vi "Do.vi"(8 "error in (no error)":errorcluster, 10 "Actor in":refnum<class "Actor.lvclass">, 11 "Load and Run Sequence Msg":refnum<class "Load and Run Sequence Msg.lvclass">) -> (0 "error out":errorcluster, 2 "Actor out":refnum<class "Actor.lvclass">)   [LabVIEW 2020, in "Sequencer.lvlib" / "Load and Run Sequence Msg.lvclass"]
doc: "This implementation loads and compiles a sequence and then enqueues it in front on the Sequencer Core."
uses:
  Load and Run Sequence Msg.lvclass
  C:/Current projects/WS/LV32.2020..HDH.ActorFramework.Core/Actor/Sequencer/Sequencer Messages/Sequencer Msg/Sequencer Msg.lvclass
  PPL/HDH.Actor Framework.Core.Actor.lvlibp/1abvi3w/vi.lib/ActorFramework/Actor/Actor.lvclass
  Sequencer/Sequencer.lvclass
  C:/Current projects/WS/PPL/HDH.Actor Framework.Core.Actor.lvlibp/1abvi3w/vi.lib/ActorFramework/Actor/Actor.lvclass
  Sequencer Msg/Sequencer Msg.lvclass/Sequencer Msg.ctl
  Load and Run Sequence Msg.lvclass/Load and Run Sequence Msg.ctl
  Batch Msg/Batch Msg.lvclass
  C:/Current projects/WS/PPL/HDH.Actor Framework.Core.Actor.lvlibp/1abvi3w/vi.lib/ActorFramework/Message/Message.lvclass
  Sequencer.lvlib
  Sequencer Msg/Sequencer Msg.lvclass
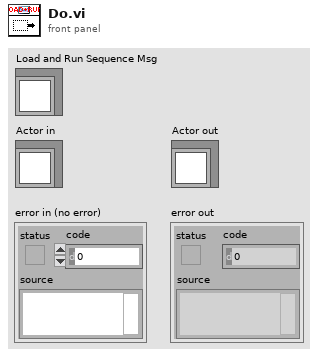
[diagram p1: front panel]
types:
  T1 = typedef "Sequencer.lvlib/Ctl_MessageListElement.ctl" = cluster{"Base Name":string, "List index":i32, "Msg path":path, "Supports DA?":bool, "Symbol":i32}
  T2 = typedef "Sequencer.lvlib/Ctl_SequenceElement.ctl" = cluster{"Message Base Name":string, "Message Path":path, "Supports Data Access?":bool, "List Symbol":i32, "Sequence Control Element Array":T3[]}
  T3 = typedef "Sequencer.lvlib/Ctl_SequenceControlElement.ctl" = cluster{"Data Override name":string, "Looped Override?":bool, "Control element":T4, "List Symbol":i32}
  T4 = typedef "HDH.Actor Framework.Core.Msg.lvlibp/Ctl_Control Element.ctl" = cluster{"Index":i32, "Label":string, "Value":variant}
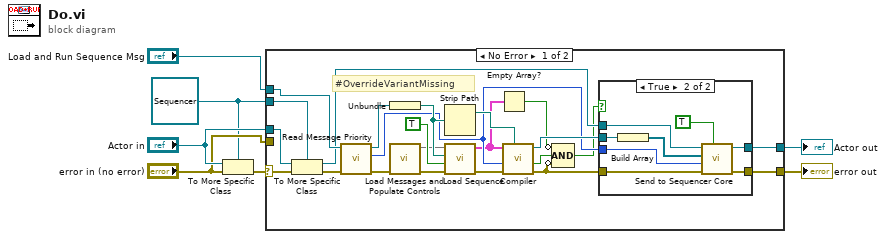
[diagram p0: block diagram]
diagram:
  w1 = refnum<class "Sequencer.lvclass"> refnum ("Sequencer.lvlib:Sequencer.lvclass")
  n1 = To More Specific Class(target class=w1, reference="Actor in", error in="error in (no error)") -> (error out=w4:errorcluster)  [unwired: 1 out]
  n2 = case shown="No Error" w4 {
    selector: w4 -> [w24 _]
    tunnel: [w17 w41] -> w7
    tunnel: [w16 w42] -> w6
    tunnel: "Actor in" -> [w22 w42]
    tunnel: "Load and Run Sequence Msg" -> [w27 _]
    tunnel: "error in (no error)" -> [_ w41]
    tunnel: w1 -> [w21 _]
    frame No Error {
      # "#OverrideVariantMissing"
      n3 = To More Specific Class(target class=w21, reference=w22, error in=w24) -> (specific class reference=w20:refnum<class "Sequencer.lvclass">, error out=w23:errorcluster)
      n4 = call "Read Message Priority.vi"("error in (no error)"=w23, "Sequencer Msg in"=w27) -> ("error out"=w10:errorcluster, "Priority"=w18:u16, "Sequencer Msg out"=w26:refnum<class "Load and Run Sequence Msg.lvclass">)  [unwired: 7 in]
      n5 = Unbundle(w26) -> (w29:path)
      n6 = call "Load Messages and Populate Controls.vi"("error in (no error)"=w10) -> ("error out"=w9:errorcluster, "Message map"=w8:map{string, T1})  [unwired: 9 in]
      n7 = Strip Path(path=w29) -> (stripped path=w28:path)  [unwired: 1 out]
      n8 = call "Load Sequence.vi"("error in (no error)"=w9, "Skip File Dialog?(F)"=TRUE, "Browse path"=w29, "Message map"=w8) -> ("error out"=w25:errorcluster, "Uncompiled Sequence out"=w15:T2[])  [unwired: 6 in]
      n9 = Empty Array?(array=w15) -> (empty?=w14:bool)
      n10 = call "Compiler.vi"("Sequence folder path"=w28, "error in (no error)"=w25, "Message Priority(Normal)"=w18, "Uncompiled sequence in"=w15) -> ("error out"=w12:errorcluster, "Success?"=w13:bool, "Batch Msg out"=w19:refnum<class "Batch Msg.lvclass">)  [unwired: 5 in]
      n11 = Compound Arithmetic op=AND(invert w14, w13, invert w12) -> (w11:bool)
      n12 = case shown="True" w11 {
        tunnel: w20 -> [w31 w40]
        tunnel: w19 -> [_ w39]
        tunnel: w18 -> [_ w36]
        tunnel: [w32 w35] -> w17
        tunnel: [w31 w34] -> w16
        tunnel: w12 -> [w32 w33]
        frame False {
        }
        frame True {
          n13 = Build Array(w39) -> (w38:refnum<class "Batch Msg.lvclass">[])
          n14 = call "Send to Sequencer Core.vi"("In Front?(F)"=TRUE, "error in (no error)"=w33, "Message Priority"=w36, "Message Array"=w38, "Sequencer in"=w40) -> ("error out"=w35:errorcluster, "Sequencer out"=w34:refnum<class "Sequencer.lvclass">)  [unwired: 5 in]
        }
      }
    }
    frame Error {
    }
  }
  "error out" <- w7
  "Actor out" <- w6
